vi "Motion_24G_xbee.vi"(0 "VISA resource name":refnum<visa-resource-name>="COM1", 1 "baud rate":u32=9600, 4 "data bits":u16=8 min=5 max=8 step=1, 5 "parity":u16(ring) items=["None", "Odd", "Even", "Mark", "Space"], 7 "stop bits":u16=10, 9 "XON Character":u8=17 format="%.0x", 14 "XOFF Character":u8=19 format="%.0x", 15 "timeout (ms)":u32=10000, 21 "End read on termination character?":bool, 24 "termination char\n(0xA = '\\n' = LF)":u8=10 format="%.0x", 25 "buffer size":u32=4096) -> ()   [LabVIEW 2015]
doc: "The Advanced Serial Read and Write example performs a Serial Port Read, a Serial Port Write, or a combination of these actions while setting some advanced serial features like buffer size, termination characters, and XON/XOFF flow control. The user selects the actions (read or write) on the front panel. If both are selected, the VI will write the data first, read the data and then close the VISA session that is opened to the port. \n\nThe parameters set for the serial port must match the parameters of the connected instrument or device. In this example, the bytes to read parameter specifies the number of bytes that the serial port reads. If there were more bytes at the port than the number specified in bytes to read, those bytes would not be read. Also, if you specify to read more bytes than the number of bytes actually read, you might receive a timeout error message.\n\nINSTRUCTIONS:\n1) Select the serial resource and configuration parameters (baud rate, data bits, parity, stop bits, flow control).\n2) Termination character can be enabled and set. Also, set the required input buffer size prior to running the example.\n3) Select the operations to be performed. \n4) Connect the serial port to your device. If no device is available, perform a loopback test by doing one of the following. Short pins 2 and 3 on a RS-232 cable or short pin 4 to pin 8 and pin 5 to pin 9 on a RS-485/422 cable. \n5) Run the VI to see the data read. (The \"read string\" will match the \"string to write\" if a loopback test was performed.)\n\nThis example exposes several advanced features that you may need for your application. Not all applications need all the features shown in this example. The input buffer size is likely an important setting that you want to control in your application. This example expands upon the flow control option for XON and XOFF, allowing the user to choose those control characters. The timeout parameter has been brought to the front panel so a user can specify the time period the VISA Read will wait for the number of bytes to read before timing out. Also, the user has several controls for the termination character, which is discussed later.\n\nNote that you can press the write and read buttons and change the bytes to read parameters on the fly, while the example is running. However, you must stop the example to change the other configuration parameters after the example has started running, and then run again.\n\nSet the I/O buffer size slightly higher the amount of data you expect to receive. This is very important for applications that don't use flow control, as you may lose characters if the receive buffer overflows.\n\nSetting the timeout period ensures that the operation returns with a timeout error if the operation cannot be performed in the specified time period. \n\nSome devices require a termination character in order to identify the end of command strings. Some devices send a termination character to signify the end of data to be read. \n\nThis example shows how you can end the Read operation once a termination character is detected in the buffer and/or append a termination character at the end of the Write data. To enable the Read to end on a termination character, use the VISA Configure Serial Port or use the VISA Properties Serial End Mode for Reads, Termination Character Enable, and Termination Character. To end the Write with a termination character, use the VISA Properties Serial End Mode for Writes, the Send End Enable, and Termination Character. In this example, the same termination character is used for both the Read and the Write. You can specify two different characters for your application, if desired.\n\nYour application may require specific characters for the XON/XOFF Flow Control. You can specify these characters with the VISA Properties Flow Control XOFF Character and Flow Control XON Character. Note that if the standard XON and XOFF characters are used, then decimal 17 and 19 are unavailable for data values. Remember that using flow control and setting an adequate buffer size allow you to prevent buffer overflows."
uses:
  <vilib>/Analysis/2dsp.llb/Complex FFT.vi
  <vilib>/Instr/_visa.llb/VISA Configure Serial Port (Instr).vi
  <vilib>/measure/madcrms.llb/Basic Averaged DC-RMS for 1 Chan.vi
  <vilib>/measure/NI_MAPro.lvlib
  <vilib>/Analysis/NI_AALPro.lvlib
panel:
  in  "Send":bool
  out "Spectrum":waveform(dbl)(graph)
  in  "Save Data":bool
  out "I/Q channels":dynamicdata(graph)
  in  "time":timestamp=timestamp(3198752888.296 s since 1904-01-01)
  in  "FFT":i32=256
  in  "stop":bool
  in  "flow control":u16(ring) items=["None"=0, "XON/XOFF"=1, "RTS/CTS"=2, "DTR/DSR"=4]
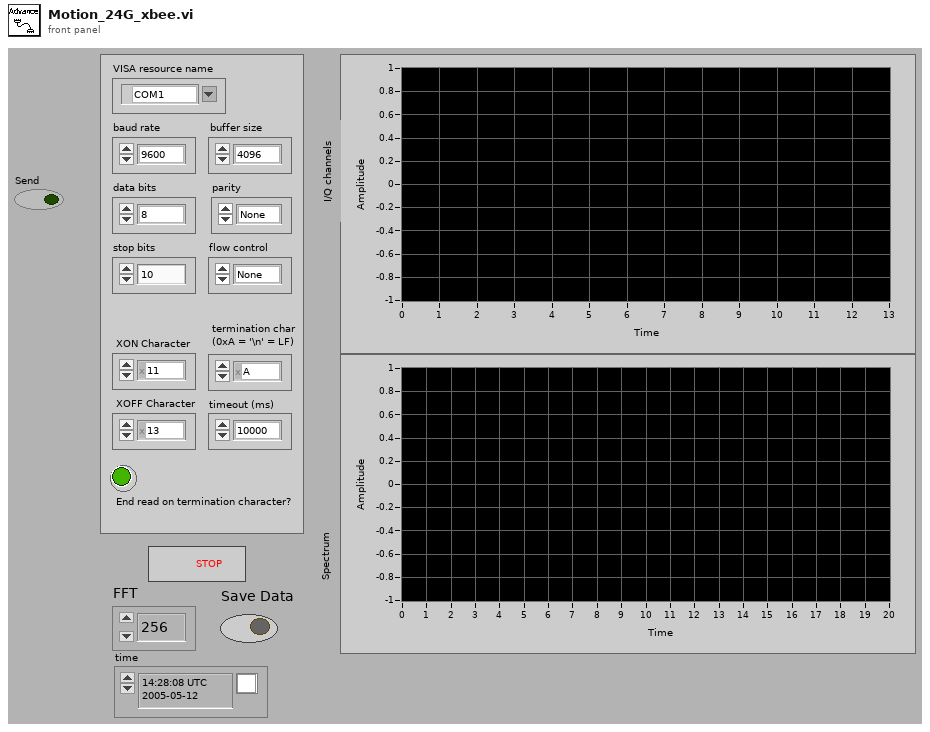
[diagram p1: front panel]
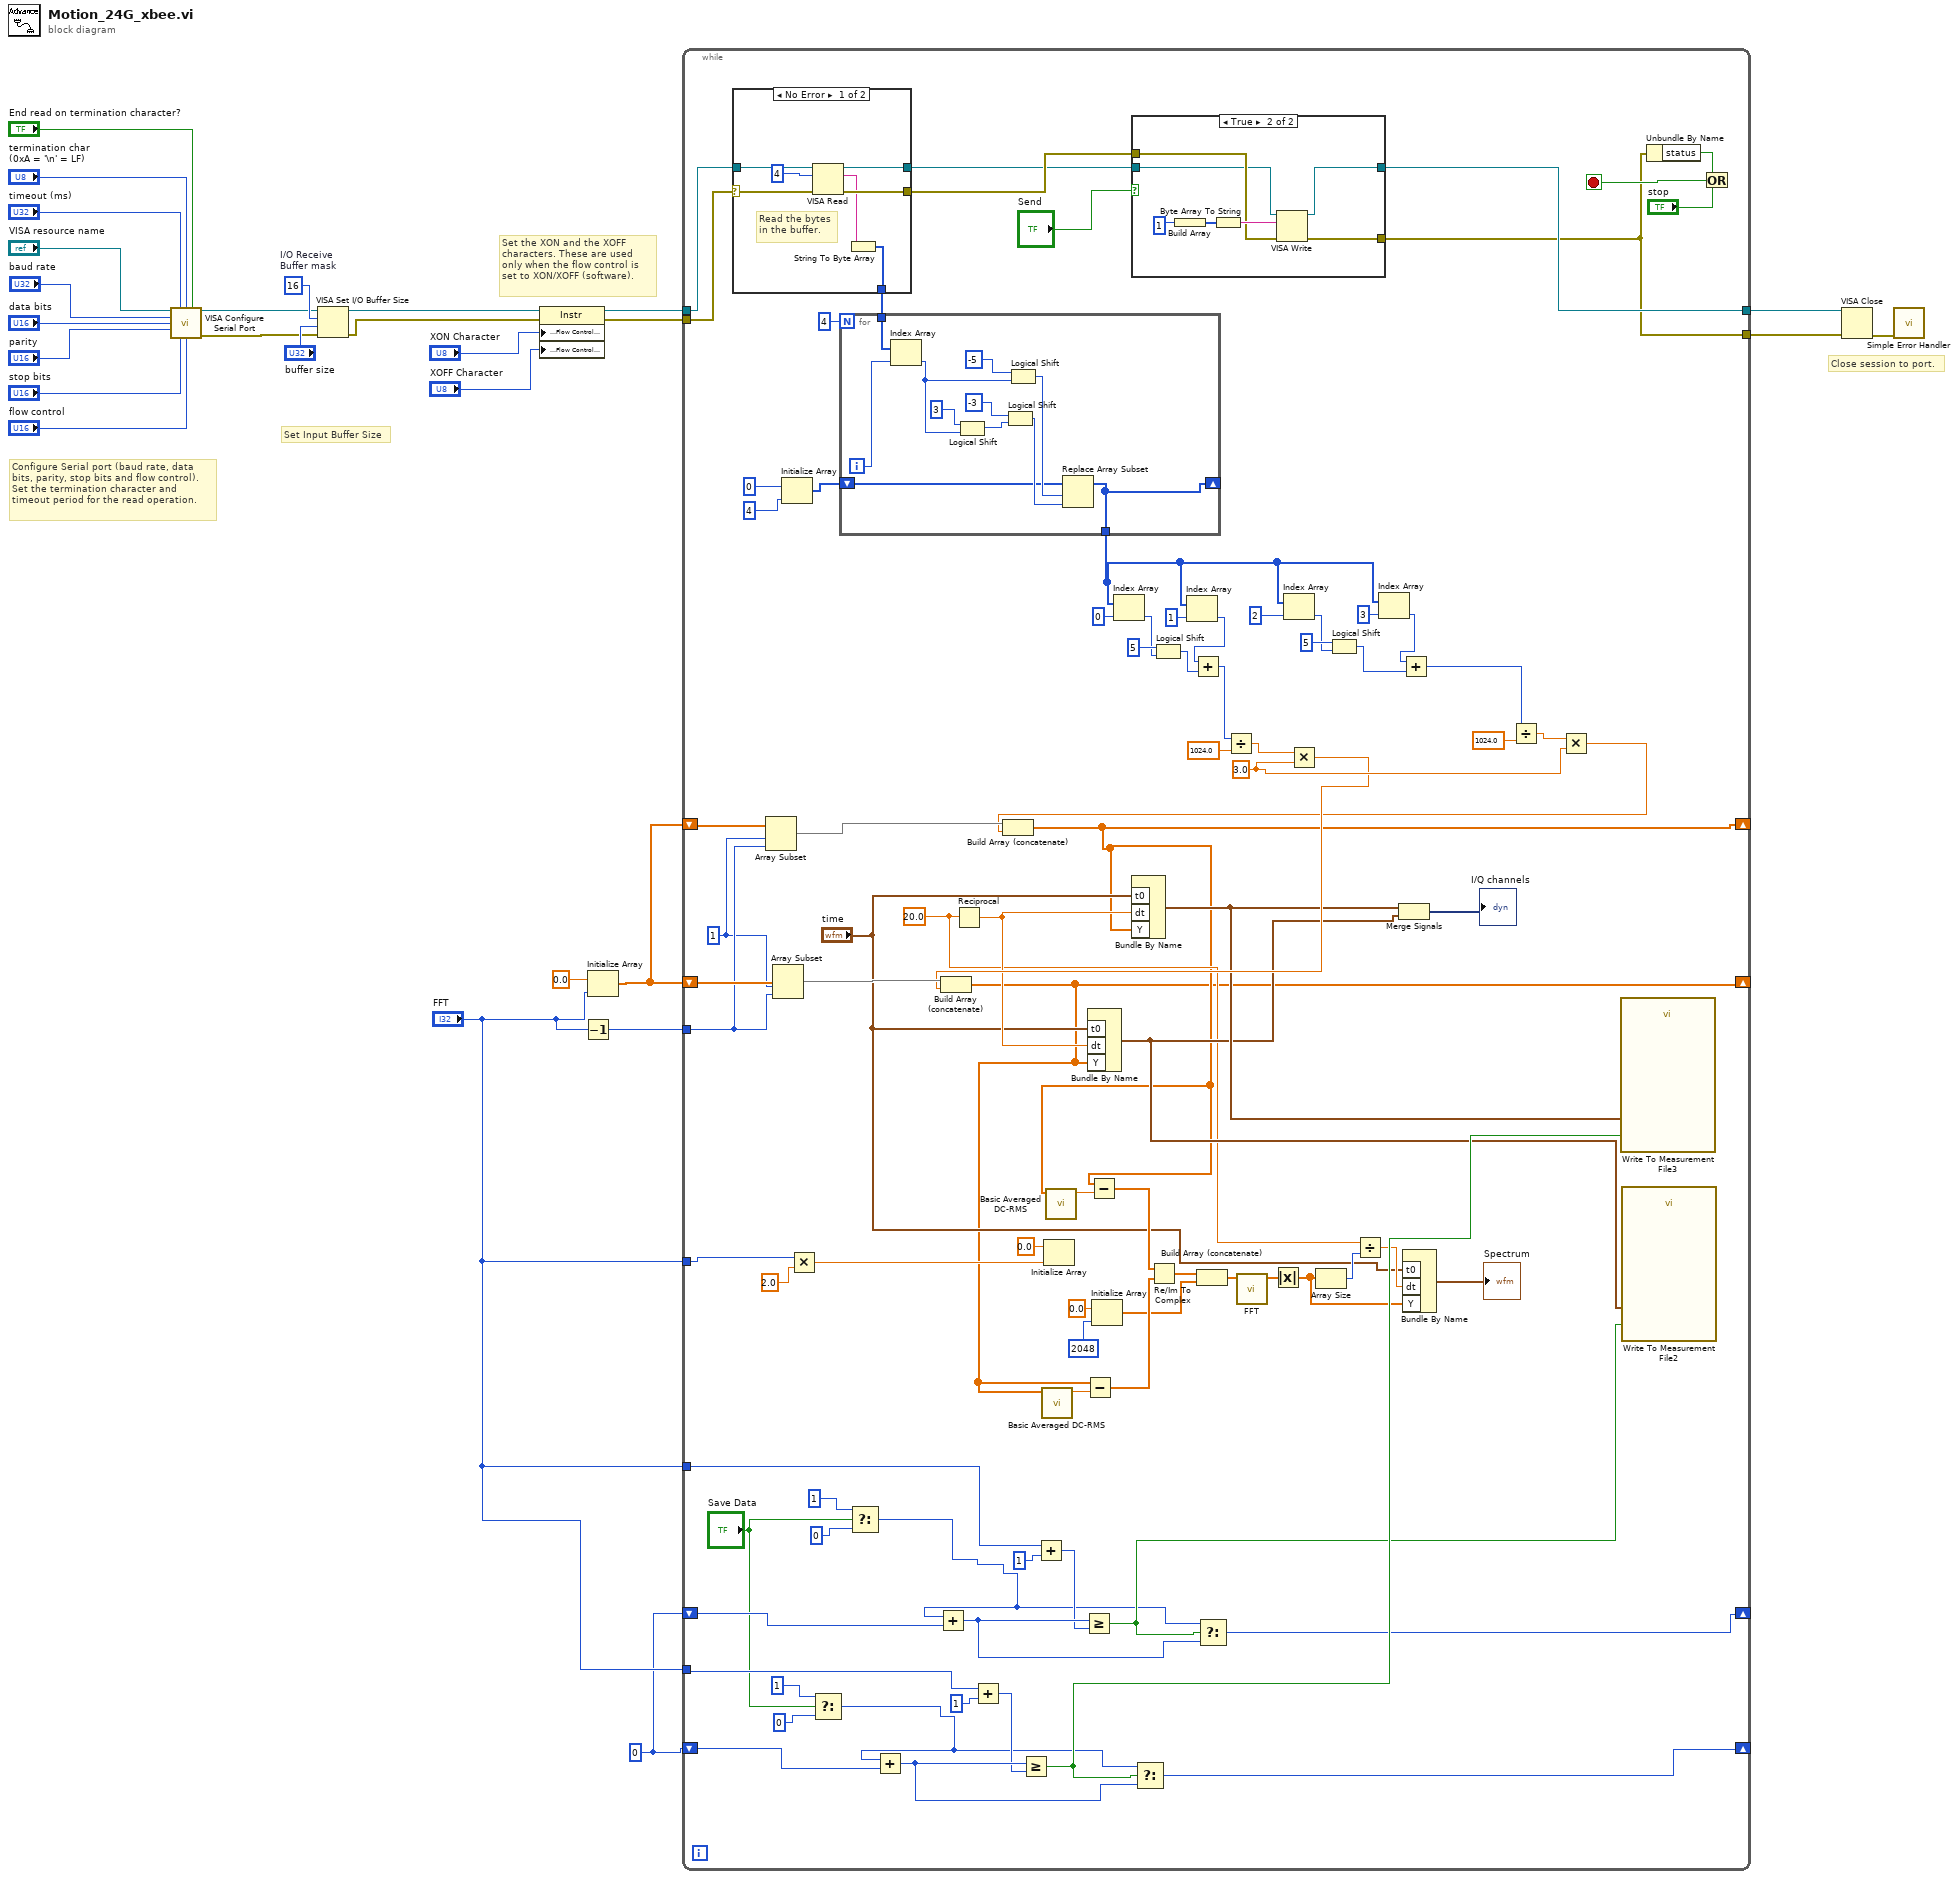
[diagram p0: block diagram]
diagram:
  w1 = 0
  w20 = u16 16  # I/O Receive Buffer mask
  # "Set the XON and the XOFF\ncharacters. These are used\nonly when the flow control is\nset to XON/XOFF (software)."
  # "Configure Serial port (baud rate, data\nbits, parity, stop bits and flow control).\nSet the termination character and\ntimeout period for the read operation."
  # "Set Input Buffer Size"
  # "Close session to port."
  n1 = call-poly "VISA Configure Serial Port"("VISA resource name"="VISA resource name", "timeout (10sec)"="timeout (ms)", "termination char\n(0xA = '\\n' = LF)"="termination char\n(0xA = '\\n' = LF)", "Enable Termination\nChar (T)"="End read on termination character?", "baud rate (9600)"="baud rate", "data bits (8)"="data bits", "parity (0:none)"="parity", "stop bits (10: 1 bit)"="stop bits", "flow control (0:none)"="flow control") -> ("VISA resource name out"=w3:refnum<visa-resource-name>, "error out"=w2:errorcluster)  [unwired: 1 in, 4 out]
  n2 = VISA Set I/O Buffer Size(VISA resource name=w3, mask (16)=w20, size (4096)="buffer size", error in (no error)=w2) -> (VISA resource name out=w16:refnum<visa-resource-name>, error out=w15:errorcluster)
  n3 = property class="Instr"(reference=w16, error in=w15, "Serial Settings:Flow Control XON Character"="XON Character", "Serial Settings:Flow Control XOFF Character"="XOFF Character") -> (reference out=w10:refnum<visa-resource-name>, error out=w12:errorcluster)
  n4 = Decrement(x="FFT") -> (x-1=w7:i32)
  n5 = Initialize Array(0.0 ("element"), "FFT") -> (w6:dbl[])
  n6 = while {
    tunnel: w12 -> [w61]
    tunnel: w10 -> [w60]
    tunnel: [w30] -> w9
    tunnel: [w29] -> w8
    tunnel: w7 -> [w98]
    shift-right: [w39] -> _
    shift-left: w6 -> [w113]
    shift-right: [w40] -> _
    shift-left: w6 -> [w99]
    shift-right: [w87] -> _
    shift-left: w1 -> [w89]
    tunnel: "FFT" -> [w83]
    tunnel: "FFT" -> [w63]
    tunnel: "FFT" -> [w73]
    shift-right: [w69] -> _
    shift-left: w1 -> [w70]
    stop <- w116 stop-if-true
    w41 = 1 ("index")
    (unwired) 0
    w90 = 3.0 ("y")
    w50 = 20.0 ("dt")
    n7 = case "Read bytes from port." shown="No Error" w61 {
      selector: w61 -> [w141 w146]
      tunnel: [w143 w146] -> w32
      tunnel: [w144 w147] -> w31
      tunnel: w60 -> [w142 w147]
      tunnel: [w139 u8[] [] ("unsigned byte array")] -> w33
      frame No Error {
        # "Read the bytes\nin the buffer."
        n8 = VISA Read(VISA resource name=w142, byte count=u32 4, error in (no error)=w141) -> (VISA resource name out=w144:refnum<visa-resource-name>, read buffer=w140:string, error out=w143:errorcluster)  [unwired: 1 out]
        n9 = String To Byte Array(string=w140) -> (unsigned byte array=w139:u8[])
      }
      frame Error {
        # "Error occurred \nreading Bytes at \nSerial Port"
      }
    }
    n10 = Array Subset(array=w99, index=w41, length=w98) -> (w100:dbl[])
    n11 = Array Subset(array=w113, index=w41, length=w98) -> (w114:dbl[])
    n12 = Initialize Array(i16 0 ("element"), 4 ("dimension size")) -> (w34:i16[])
    n13 = Multiply(x=w63, y=2.0 ("dt")) -> (x*y=w64:dbl)
    n14 = Select(t=1, s="Save Data", f=0) -> (s? t:f=w37:i32)
    n15 = for {
      N: 4 -> [_]
      tunnel: w33 -> [w132]
      tunnel: [w127] -> w42
      shift-right: [w127] -> _
      shift-left: w34 -> [w128]
      i -> [w131]
      n16 = Index Array(array=w132, index=w131) -> (element=w135:u8)
      n17 = Logical Shift(y=i8 3, x=w135) -> (x << y=w134:u8)
      n18 = Logical Shift(y=i8 -3, x=w134) -> (x << y=w129:u8)
      n19 = Logical Shift(y=i8 -5, x=w135) -> (x << y=w130:u8)
      n20 = Replace Array Subset(array=w128, new element=w129, index=w130) -> (w127:i16[])
    }
    n21 = Select(t=1, s="Save Data", f=0) -> (s? t:f=w38:i32)
    n22 = Add(x=w37, y=w89) -> (x+y=w88:i32)
    n23 = Add(x=w38, y=w70) -> (x+y=w76:i32)
    n24 = Reciprocal(x=w50) -> (1/x=w79:dbl)
    n25 = Add(x=w83, y=1) -> (x+y=w84:i32)
    n26 = Greater Or Equal?(x=w88, y=w84) -> (x >= y?=w86:bool)
    n27 = Add(x=w73, y=1) -> (x+y=w74:i32)
    n28 = Initialize Array(0.0 ("element"), w64) -> ()  [unwired: 1 out]
    n29 = Greater Or Equal?(x=w76, y=w74) -> (x >= y?=w65:bool)
    n30 = Initialize Array(0.0 ("element"), 2048 ("dimension size")) -> (w54:dbl[])
    n31 = Index Array(array=w42, index=0) -> (element=w107:i16)
    n32 = case shown="True" "Send" {
      tunnel: w32 -> [w119 w125]
      tunnel: w31 -> [w118 w124]
      tunnel: [w118 w123] -> w30
      tunnel: [w119 w122] -> w29
      frame False {
      }
      frame True {
        n33 = Build Array(u8 1 ("unsigned byte array")) -> (w120:u8[])
        n34 = Byte Array To String(unsigned byte array=w120) -> (string=w126:string)
        n35 = VISA Write(VISA resource name=w124, write buffer=w126, error in (no error)=w125) -> (VISA resource name out=w123:refnum<visa-resource-name>, error out=w122:errorcluster)  [unwired: 1 out]
      }
    }
    n36 = Select(t=w37, s=w86, f=w88) -> (s? t:f=w87:i32)
    n37 = Logical Shift(y=i16 5, x=w107) -> (x << y=w103:i16)
    n38 = Index Array(array=w42, index=1) -> (element=w104:i16)
    n39 = Add(x=w104, y=w103) -> (x+y=w45:i16)
    n40 = Select(t=w38, s=w65, f=w76) -> (s? t:f=w69:i32)
    n41 = Divide(x=w45, y=1024.0) -> (x/y=w96:dbl)
    n42 = Index Array(array=w42, index=2) -> (element=w105:i16)
    n43 = Multiply(x=w96, y=w90) -> (x*y=w81:dbl)
    n44 = Build Array (concatenate)(w114, w81) -> (w39:dbl[])
    n45 = call-poly <vilib>:"Basic Averaged DC-RMS.vi"("signal in"=w39) -> ("DC value"=w91:dbl)  [unwired: 4 in, 6 out]
    n46 = Subtract(x=w39, y=w91) -> (x-y=w58:dbl[])
    n47 = Bundle By Name ("Build Waveform")("t0"="time", "dt"=w79, "Y"=w39) -> (w66:waveform(dbl))  [unwired: 1 out]
    n48 = Logical Shift(y=i16 5, x=w105) -> (x << y=w101:i16)
    n49 = Index Array(array=w42, index=3) -> (element=w102:i16)
    n50 = Add(x=w102, y=w101) -> (x+y=w44:i16)
    n51 = Divide(x=w44, y=1024.0) -> (x/y=w94:dbl)
    n52 = Multiply(x=w94, y=w90) -> (x*y=w80:dbl)
    n53 = Build Array (concatenate)(w100, w80) -> (w40:dbl[])
    n54 = call-poly <vilib>:"Basic Averaged DC-RMS.vi"("signal in"=w40) -> ("DC value"=w92:dbl)  [unwired: 4 in, 6 out]
    n55 = Subtract(x=w40, y=w92) -> (x-y=w59:dbl[])
    n56 = Bundle By Name ("Build Waveform")("t0"="time", "dt"=w79, "Y"=w40) -> (w67:waveform(dbl))  [unwired: 1 out]
    n57 = Re/Im To Complex(1:w58, 2:w59) -> (0:w53:cdb[])
    n58 = Build Array (concatenate)(w53, w54) -> (w55:cdb[])
    n59 = call-poly <vilib>:"FFT.vi"("X"=w55) -> ("FFT {X}"=w51:cdb[])  [unwired: 2 in, 8 out]
    n60 = Absolute Value(x=w51) -> (abs(x)=w49:dbl[])
    n61 = Array Size(array=w49) -> (size(s)=w52:i32)
    n62 = Divide(x=w50, y=w52) -> (x/y=w48:dbl)
    n63 = Merge Signals(w67, w66) -> (→"I/Q channels":dynamicdata)
    n64 = Bundle By Name("t0"="time", "dt"=w48, "Y"=w49) -> (→"Spectrum":waveform(dbl))  [unwired: 1 out]
    n65 = call "Write To Measurement File3"("Signals"=w67, "Enable"=w86) -> ()  [unwired: 15 in, 3 out]
    n66 = call "Write To Measurement File2"("Signals"=w66, "Enable"=w65) -> ()  [unwired: 15 in, 3 out]
    n67 = Unbundle By Name(w29) -> ("status"=w117:bool)
    n68 = Or(x=w117, y="stop") -> (x .or. y?=w116:bool)
  }
  n69 = VISA Close(VISA resource name=w9, error in (no error)=w8) -> (error out=w25:errorcluster)
  n70 = call <vilib>:"Simple Error Handler.vi"("error in (no error)"=w25) -> ()  [unwired: 1 in, 8 out]
